vi "SetShifterNotes.vi"(7 "LabVIEW Web Service Request":refnum<class "Web Request.lvclass">) -> ()   [LabVIEW 2018]
uses:
  <vilib>/wsapi/Web Request.lvclass
  CAEN globals.vi
panel:
  in  "error in (no error)":errorcluster
  # "Use the Web Service Request input terminal to call the VIs on the Web Services palette. Do not remove it from the connector pane unless you don't need access to the palette."
  # "Each additional control wired to the connector pane will be available as an input in the URL. To include an indicator in terminal-mode output (the default setting), it must also be wired to the connector pane."
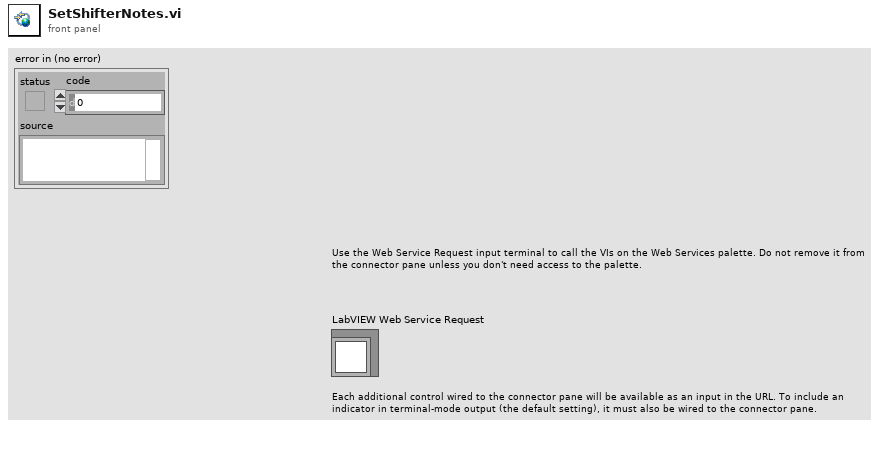
[diagram p1: front panel]
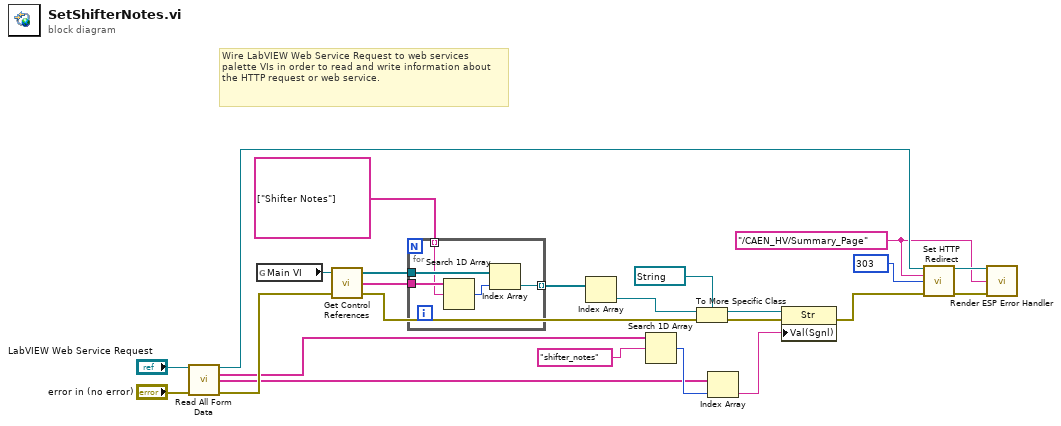
[diagram p0: block diagram]
diagram:
  w3 = "/CAEN_HV/Summary_Page" ("redirect URL")
  w19 = 303 items=["100"=100, "101"=101, "200"=200, "201"=201, "202"=202, "203"=203, "204"=204, "205"=205, "206"=206, "300"=300, "301"=301, "302"=302, "303"=303, "304"=304, "305"=305, "306"=306, "307"=307, "400"=400, "401"=401, "402"=402, "403"=403, "404"=404, "405"=405, "406"=406, "407"=407, "408"=408, "409"=409, "410"=410, "411"=411, "412"=412, "413"=413, "414"=414, "415"=415, "416"=416, "417"=417, "500"=500, "501"=501, "502"=502, "503"=503, "504"=504, "505"=505] ("response code (307)")
  # "Wire LabVIEW Web Service Request to web services palette VIs in order to read and write information about the HTTP request or web service."
  n1 = call <vilib>:"Read All Form Data.vi"("LabVIEW Web Service Request"="LabVIEW Web Service Request", "error in (no error)"="error in (no error)") -> ("LabVIEW Web Service Request out"=w10:refnum<class "Web Request.lvclass">, "Key"=w6:string[], "Value"=w7:string[], "error out"=w11:errorcluster)  [unwired: 9 in, 1 out]
  n2 = global read "CAEN globals.vi" "Main VI"() -> (w24:refnum<vi>)
  n3 = call "Get Control References.vi"("error in"=w11, "This vi"=w24) -> ("error out"=w13:errorcluster, "Control Names"=w23:string[], "Controls[]"=w22:refnum<vi>[])  [unwired: 1 in]
  n4 = for {
    tunnel: w23 -> [w29]
    tunnel: w22 -> [w28]
    tunnel: [w26] -> w8 mode=indexing
    tunnel: string[] ["Shifter Notes"] ("Control Names") -> [w25] mode=indexing
    n5 = Search 1D Array(1D array=w29, element=w25) -> (index of element=w27:i32)  [unwired: 1 in]
    n6 = Index Array(array=w28, index=w27) -> (element=w26:refnum<vi>)
  }
  n7 = Index Array(array=w8) -> (element=w4:refnum<vi>)  [unwired: 1 in]
  n8 = Search 1D Array(1D array=w6, element="shifter_notes") -> (index of element=w15:i32)  [unwired: 1 in]
  n9 = To More Specific Class(target class=refnum<vi> refnum ("element"), reference=w4, error in=w13) -> (specific class reference=w20:refnum<vi>, error out=w21:errorcluster)
  n10 = Index Array(array=w7, index=w15) -> (element=w1:string)
  n11 = property class="Str"(reference=w20, error in=w21, "Val(Sgnl)"=w1) -> (error out=w2:errorcluster)  [unwired: 1 out]
  n12 = call <vilib>:"Set HTTP Redirect.vi"("LabVIEW Web Service Request"=w10, "redirect URL"=w3, "response code (307)"=w19, "error in (no error)"=w2) -> ("LabVIEW Web Service Request out"=w17:refnum<class "Web Request.lvclass">, "error out"=w18:errorcluster)  [unwired: 10 in]
  n13 = call "Render ESP Error Handler.vi"("LabVIEW Web Service Request"=w17, "Link"=w3, "error in (no error)"=w18) -> ()  [unwired: 11 in, 2 out]
